vi "niDTS GNSS RF Test Initialize.vi"(0 "Dut Reference":T2, 5 "SystemTechnologyCatalog":refnum<class "niDTS SystemTechnologyCatalog.lvclass">, 7 "SystemDut":refnum<class "niDTS SystemDut.lvclass">, 9 "Logger Reference":T1, 11 "error in (no error)":errorcluster) -> (4 "Dummy Test Handle out":T3, 15 "error out":errorcluster)   [LabVIEW 2014, in "niDTS GNSS.lvlib"]
uses:
  niDTS GNSS.lvlib
  Includes/niDTS GNSS RF Test INC Handle.ctl
  Objects/BASE_class/niDTS GNSS RF Test.lvclass
  Framework/Dut/Includes/niDTS Dut INC Handle.ctl
  Framework/Dut/Objects/BASE_class/niDTS Dut.lvclass
  Framework/Logger/Includes/niDTS Logger INC Handle.ctl
  Framework/Logger/Objects/BASE_class/niDTS Logger.lvclass
  TestStand/Station/Objects/SystemTechnologyCatalog/niDTS SystemTechnologyCatalog.lvclass
  TestStand/Station/Objects/SystemDut/niDTS SystemDut.lvclass
  TestStand/niDTS TestStand.lvlib
  Framework/niDTS Framework.lvlib
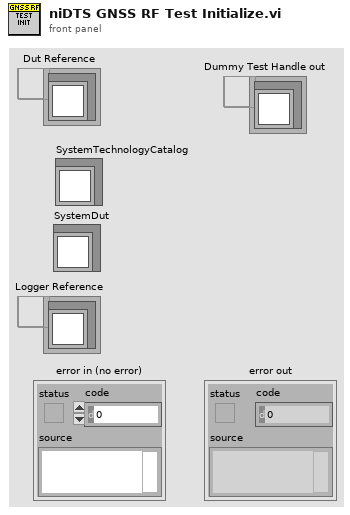
[diagram p1: front panel]
types:
  T1 = typedef "niDTS Framework.lvlib/niDTS Logger INC Handle.ctl" = refnum<data-value>
  T2 = typedef "niDTS Framework.lvlib/niDTS Dut INC Handle.ctl" = refnum<data-value>
  T3 = typedef "niDTS GNSS.lvlib/niDTS GNSS RF Test INC Handle.ctl" = refnum<data-value>
  T4 = typedef "niDTS TestStand.lvlib/niDTS TestStep INC Handle.ctl" = refnum<data-value>
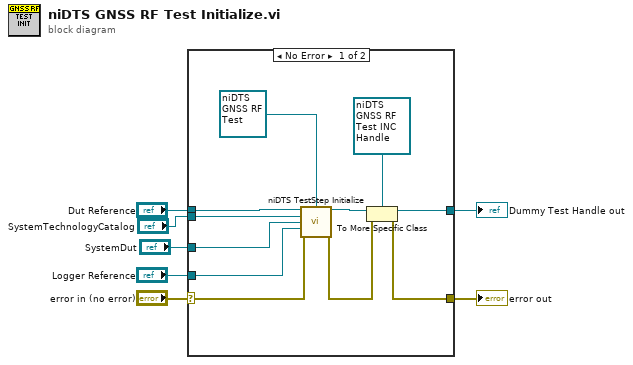
[diagram p0: block diagram]
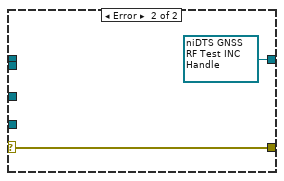
[diagram p2: hidden frame]
diagram:
  n1 = case shown="No Error" "error in (no error)" {
    selector: "error in (no error)" -> [w8 w20]
    tunnel: "Dut Reference" -> [w18 _]
    tunnel: [w16 T3 refnum ("Template Tx Test Handle")] -> w6
    tunnel: [w14 w20] -> w5
    tunnel: "Logger Reference" -> [w13 _]
    tunnel: "SystemTechnologyCatalog" -> [w10 _]
    tunnel: "SystemDut" -> [w9 _]
    frame No Error {
      n2 = call "niDTS TestStep Initialize.vi"("Dut Handle"=w18, "Test Type"=refnum<class "niDTS GNSS RF Test.lvclass"> refnum ("Dummy Test.lvlib:Dummy Test.lvclass"), "SystemTechnologyCatalog"=w10, "SystemDut"=w9, "Logger Reference"=w13, "error in (no error)"=w8) -> ("Test Handle out"=w17:T4, "error out"=w15:errorcluster)  [unwired: 8 in]
      n3 = To More Specific Class(target class=T3 refnum ("Template Tx Test Handle"), reference=w17, error in=w15) -> (specific class reference=w16:T3, error out=w14:errorcluster)
    }
    frame Error {
    }
  }
  "error out" <- w5
  "Dummy Test Handle out" <- w6
